vi "get_value_for_boolean.vi"(8 "error in (no error)":errorcluster, 11 "Value in":refnum<class "Value.lvclass">) -> (0 "error out":errorcluster, 3 "boolean_value":bool)   [LabVIEW 2020, in "toml_edit.lvlib" / "Value.lvclass"]
uses:
  Value.lvclass
  value_type--enum.ctl
  Value.lvclass/Value.ctl
  dragon_toml_64.dll
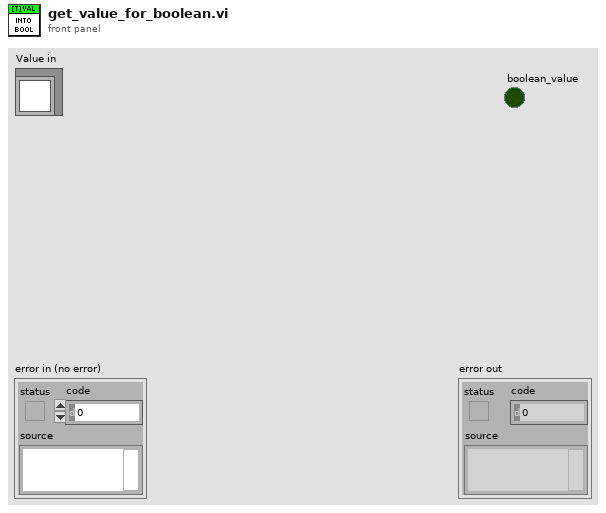
[diagram p1: front panel]
types:
  T1 = typedef "toml_edit.lvlib/Value.lvclass/value_type--enum.ctl" = enum16{"Unknown", "String", "Integer", "Float", "Boolean", "Datetime", "Array", "InlineTable"}
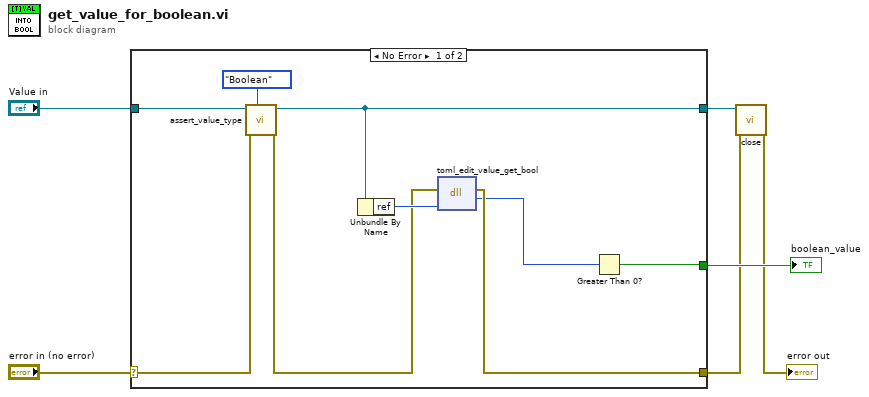
[diagram p0: block diagram]
diagram:
  n1 = case shown="No Error" "error in (no error)" {
    selector: "error in (no error)" -> [w11 w16]
    tunnel: "Value in" -> [w12 w17]
    tunnel: [w8 _] -> w4
    tunnel: [w15 w16] -> w3
    tunnel: [w9 w17] -> w2
    frame No Error {
      n2 = call "assert_value_type.vi"("value_type"=value_type--enum."Boolean", "error in (no error)"=w11, "Value in"=w12) -> ("error out"=w10:errorcluster, "Value out"=w9:refnum<class "Value.lvclass">)  [unwired: 7 in]
      n3 = Unbundle By Name(w9) -> ("ref"=w14:u64)
      n4 = dll-call lib="C:/Projects/labview-project-load-tools/source/submodules/toml-edit-labview/lv_src/dragon_toml_*.*" fn="toml_edit_value_get_bool"(error in=w10, "item_ref"=w14) -> (error out=w15:errorcluster, "boolean"=w7:i8)  [unwired: 3 in, 1 out]
      n5 = Greater Than 0?(x=w7) -> (x > 0?=w8:bool)
    }
    frame Error {
    }
  }
  "boolean_value" <- w4
  n6 = call "close.vi"("error in (no error)"=w3, "Value in"=w2) -> ("error out"=→"error out":errorcluster)  [unwired: 9 in]
